vi "test_VISA Initialize.vi"(8 "error in (no error)":errorcluster, 11 "TestCase in":refnum<class "Instrument Addon Serial Protocols Unit Tests.lvclass">) -> (0 "error out":errorcluster, 3 "TestCase out":refnum<class "Instrument Addon Serial Protocols Unit Tests.lvclass">)   [LabVIEW 2020, in "Instrument Addon Serial Protocols Unit Tests.lvclass"]
uses:
  Instrument Addon Serial Protocols Unit Tests.lvclass
  VISA/VISA.lvclass
  C:/Users/nitest/Desktop/Git 2020/niveristand-instrument-addon-classes/Source/Protocols/Protocol Parent/Protocol Parent.lvclass
  Listener/Listener.lvclass
  Listener/ListenerClassControls/Operation.ctl
  Listener/Listener.lvclass/Listener.ctl
  VISA/VISA.lvclass/VISA.ctl
  <vilib>/addons/_JKI Toolkits/VI Tester/TestCase.llb/TestCase.lvclass
  C:/Program Files (x86)/National Instruments/LabVIEW 2020/vi.lib/addons/_JKI Toolkits/VI Tester/TestCase.llb/TestCase.lvclass
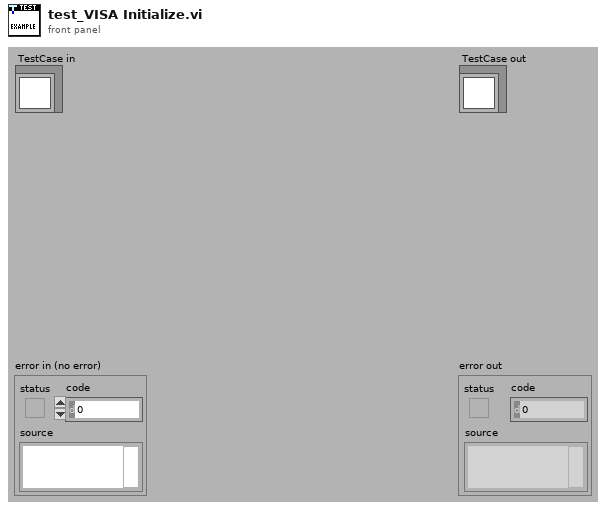
[diagram p1: front panel]
types:
  T1 = typedef "Listener.lvclass/Operation.ctl" = enum16{"Read", "Write"}
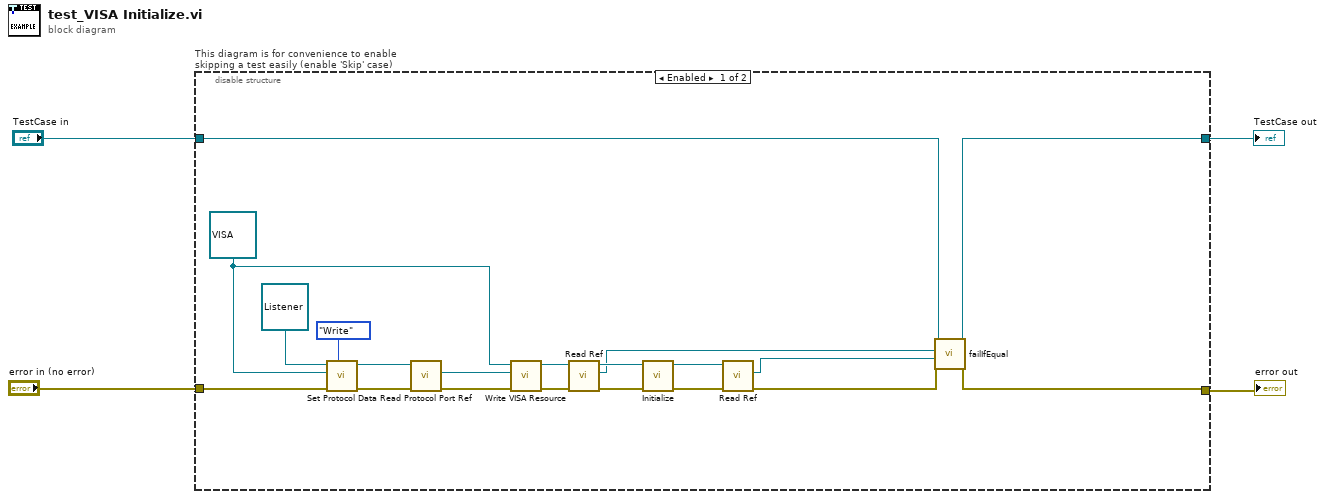
[diagram p0: block diagram]
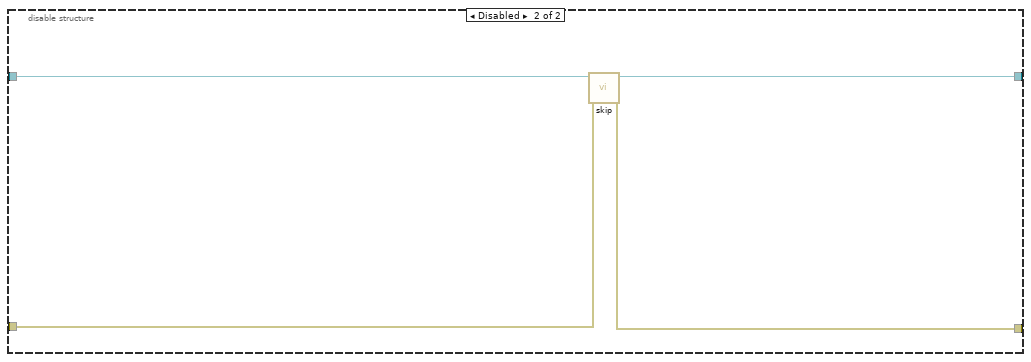
[diagram p2: hidden frame]
diagram:
  n1 = disable-structure "This diagram is for convenience to enable skipping a test easily (enable 'Skip' case)" shown="Enabled" {
    disable-tunnel: "TestCase in" -> [w24 w28]
    disable-tunnel: [w23 w26] -> w1
    disable-tunnel: [w22 w27] -> w3
    disable-tunnel: "error in (no error)" -> [w19 w25]
    frame Enabled {
      w18 = refnum<class "VISA.lvclass"> refnum ("Protocols.lvlib:VISA.lvclass")
      n2 = call "Set Protocol Data.vi"("Operation"=Operation."Write", "error in (no error)"=w19, "Protocols.lvlib:Protocol Parent.lvclass"=w18, "Listener In.lvclass"=refnum<class "Listener.lvclass"> refnum ("Listener.lvclass")) -> ("error out"=w7:errorcluster, "Listener Out.lvclass"=w8:refnum<class "Listener.lvclass">)  [unwired: 6 in]
      n3 = call "Read Protocol Port Ref.vi"("error in (no error)"=w7, "Listener in"=w8) -> ("error out"=w6:errorcluster, "Protocol Port Ref"=w5:refnum<visa-resource-name>)  [unwired: 7 in, 1 out]
      n4 = call "Write VISA Resource.vi"("error in (no error)"=w6, "VISA Resource"=w5, "VISA in"=w18) -> ("error out"=w17:errorcluster, "VISA out"=w16:refnum<class "VISA.lvclass">)  [unwired: 7 in]
      n5 = call "Read Ref.vi"("error in (no error)"=w17, "VISA in"=w16) -> ("error out"=w15:errorcluster, "Ref"=w13:refnum<visa-resource-name>, "VISA out"=w14:refnum<class "VISA.lvclass">)  [unwired: 7 in]
      n6 = call-dynamic "Initialize.vi"("error in (no error)"=w15, "VISA in"=w14) -> ("error out"=w12:errorcluster, "VISA out"=w11:refnum<class "VISA.lvclass">)  [unwired: 8 in]
      n7 = call "Read Ref.vi"("error in (no error)"=w12, "VISA in"=w11) -> ("error out"=w9:errorcluster, "Ref"=w10:refnum<visa-resource-name>)  [unwired: 7 in, 1 out]
      n8 = call-dynamic "failIfEqual.vi"("error in (no error)"=w9, "y"=w10, "x"=w13, "TestCase in"=w24) -> ("error out"=w22:errorcluster, "TestCase out"=w23:refnum<class "Instrument Addon Serial Protocols Unit Tests.lvclass">)  [unwired: 6 in]
    }
    frame Disabled {
      # "skip test result while test is under development"
      n9 = call <vilib>:"skip.vi"("error in (no error)"=w25, "TestCase in"=w28) -> ("error out"=w27:errorcluster, "TestCase out"=w26:refnum<class "Instrument Addon Serial Protocols Unit Tests.lvclass">)  [unwired: 8 in]
    }
  }
  "error out" <- w3
  "TestCase out" <- w1
